vi "apply.graphic.filter.vi"(8 "error in (no error)":errorcluster, 10 "selection filter":T1={"Volume Type"={"Ongoing"=TRUE, "Limited Series"=TRUE, "Annuals"=TRUE, "One Shots"=TRUE, "Reference/Reprints"=TRUE, "Digital"=TRUE}, "team"=[], "characters"=[], "storyArcs"=[], "Plot End"=timestamp(0 s since 1904-01-01), "Plot Start"=timestamp(0 s since 1904-01-01), "title"=[], "colors"={"ongoing"=0, "Limited Series"=0, "Annuals"=0, "One Shots"=0, "Reprints"=0, "Digital"=0}, "concept"=[], "show all"=FALSE, "Search by Title"=enum."AND", "pub ids"=[]}, 11 "manager_daemon in":refnum<class "manager_daemon.lvclass">) -> (0 "error out":errorcluster, 3 "manager_daemon out":refnum<class "manager_daemon.lvclass">)   [LabVIEW 2024, in "manager_daemon.lvclass"]
uses:
  manager_daemon.lvclass
  TypeDefs/graphic.filter--cluster.ctl
  Graphic_UI/typedefs/volume.type.colors--cluster.ctl
  manager_daemon.lvclass/manager_daemon.ctl
  TypeDefs/issue.display--cluster.ctl
  CV_Shared_Library/volume.object--cluster.ctl
  CV_Shared_Library/volume.type--enum.ctl
  e2a5ae27-bb6a-44f0-90d7-e473ed9168d5.vi
  CV_Shared_Library/CV_Shared_Library.lvlib
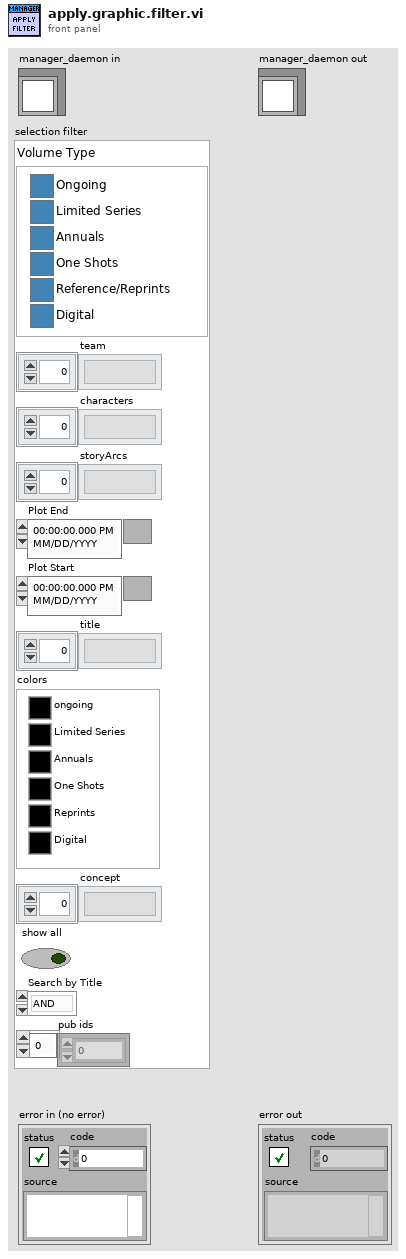
[diagram p1: front panel]
types:
  T1 = typedef "CV_Shared_Library.lvlib/graphic.filter--cluster.ctl" = cluster{"Volume Type":cluster{"Ongoing":bool, "Limited Series":bool, "Annuals":bool, "One Shots":bool, "Reference/Reprints":bool, "Digital":bool}, "team":string[], "characters":string[], "storyArcs":string[], "Plot End":timestamp, "Plot Start":timestamp, "title":string[], "colors":T2, "concept":string[], "show all":bool, "Search by Title":enum32{"AND", "OR"}, "pub ids":i32[]}
  T2 = typedef "volume.type.colors--cluster.ctl" = cluster{"ongoing":u32, "Limited Series":u32, "Annuals":u32, "One Shots":u32, "Reprints":u32, "Digital":u32}
  T3 = cluster{"Ongoing":bool, "Limited Series":bool, "Annuals":bool, "One Shots":bool, "Reference/Reprints":bool, "Digital":bool}
  T4 = typedef "manager_daemon.lvclass/IssueData--clustrer.ctl" = cluster{"cover_date":timestamp, "cv_id":string, "name":string, "sortable_name":string, "issue_number":string, "deck":string, "description":string, "volume id":i32, "store_date":timestamp, "date_last_updated":timestamp, "site_detail_url":string, "cover_url":string, "source_path":path, "in_collection":bool, "display_date":timestamp}
  T5 = typedef "manager_daemon.lvclass/sub-map--map.ctl" = map{string, T6}
  T6 = typedef "manager_daemon.lvclass/SubData--cluster.ctl" = cluster{"id":i32, "issues":set{i32}}
  T7 = typedef "manager_daemon.lvclass/VolumeData--cluster.ctl" = cluster{"name":string, "sortable_name":string, "aliases":string[], "description":string, "site_detail_url":string, "count_of_issues":i32, "start_year":i32, "publisher_id":i32, "issue_ids":i32[], "date_last_updated":timestamp, "volume":i32, "cv_id":string, "volume type":T8, "source_path":path}
  T8 = typedef "CV_Shared_Library.lvlib/volume.type--enum.ctl" = enum16{"Ongoing", "Limited Series", "Annual", "One Shot", "Reprint/Document", "Digital"}
  T9 = typedef "CV_Shared_Library.lvlib/volume.object--cluster.ctl" = cluster{"start date":timestamp, "end date":timestamp, "sortable_name":string, "color":u32, "volume type":T8, "issues":T10[]}
  T10 = typedef "CV_Shared_Library.lvlib/issue.display--cluster.ctl" = cluster{"cover_date":timestamp, "id":i32, "number":string, "fill":bool, "hilight":bool}
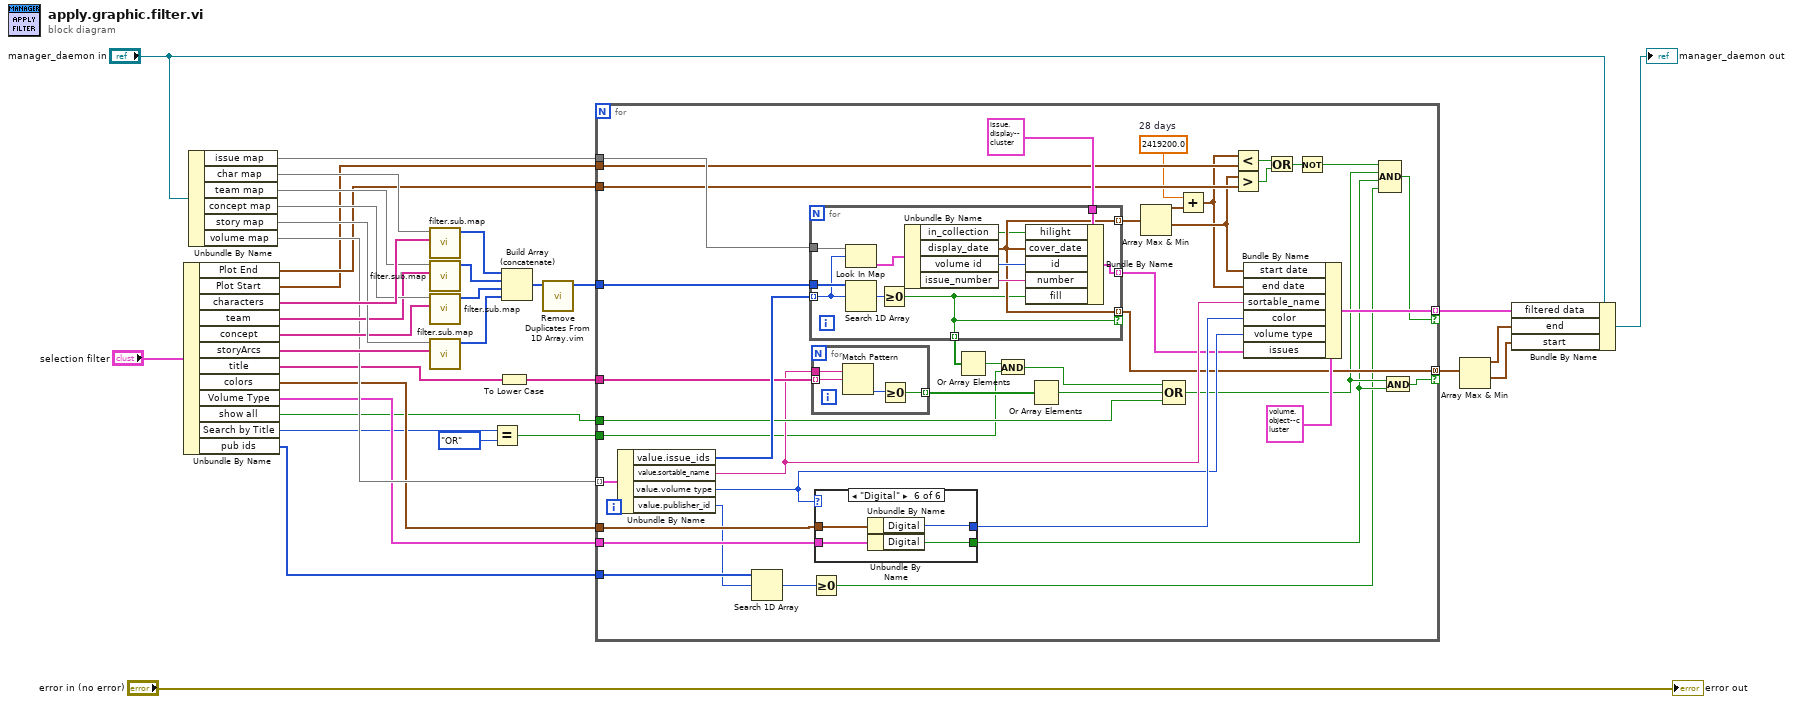
[diagram p0: block diagram]
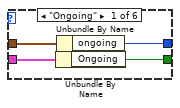
[diagram p2: hidden frame]
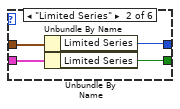
[diagram p3: hidden frame]
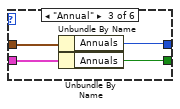
[diagram p4: hidden frame]
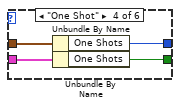
[diagram p5: hidden frame]
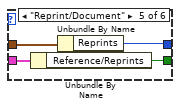
[diagram p6: hidden frame]
diagram:
  n1 = Unbundle By Name("selection filter") -> ("Plot End"=w14:timestamp, "Plot Start"=w13:timestamp, "characters"=w33:string[], "team"=w29:string[], "concept"=w28:string[], "storyArcs"=w27:string[], "title"=w19:string[], "colors"=w16:T2, "Volume Type"=w15:T3, "show all"=w12:bool, "Search by Title"=w7:enum32{"AND", "OR"}, "pub ids"=w1:i32[])
  n2 = Unbundle By Name("manager_daemon in") -> ("issue map"=w17:map{i32, T4}, "char map"=w34:T5, "team map"=w32:T5, "concept map"=w31:T5, "story map"=w30:T5, "volume map"=w26:map{i32, T7})
  n3 = call "filter.sub.map"("filter"=w33, "sub-map"=w34) -> ("issues"=w25:i32[])  [unwired: 9 in]
  n4 = call "filter.sub.map"("filter"=w29, "sub-map"=w32) -> ("issues"=w24:i32[])  [unwired: 9 in]
  n5 = call "filter.sub.map"("filter"=w28, "sub-map"=w31) -> ("issues"=w23:i32[])  [unwired: 9 in]
  n6 = call "filter.sub.map"("filter"=w27, "sub-map"=w30) -> ("issues"=w22:i32[])  [unwired: 9 in]
  n7 = Equal?(x=w7, y=enum32{"AND", "OR"}."OR") -> (x = y?=w5:bool)
  n8 = To Lower Case(string=w19) -> (all lower case string=w18:string[])
  n9 = Build Array (concatenate)(w25, w24, w23, w22) -> (w21:i32[])
  n10 = call "Remove Duplicates From 1D Array.vim"("array"=w21) -> ("array with duplicates removed"=w20:i32[])  [unwired: 10 in]
  n11 = for {
    tunnel: w26 -> [w76] mode=indexing
    tunnel: w20 -> [w74]
    tunnel: w18 -> [w72]
    tunnel: w17 -> [w73]
    tunnel: w16 -> [w69]
    tunnel: w15 -> [w68]
    tunnel: w14 -> [w64]
    tunnel: w13 -> [w65]
    tunnel: w12 -> [w60]
    tunnel: [w51] -> w9 mode=indexing if=w50
    tunnel: w5 -> [w45]
    tunnel: [w43] -> w4 mode=concatenating if=w42
    tunnel: w1 -> [w39]
    w49 = 2419200.0  # 28 days
    n12 = Unbundle By Name(w76) -> ("value.issue_ids"=w75:i32[], "value.sortable_name"=w55:string, "value.volume type"=w53:T8, "value.publisher_id"=w38:i32)
    n13 = Search 1D Array(1D array=w39, element=w38) -> (index of element=w37:i32)  [unwired: 1 in]
    n14 = for {
      tunnel: w75 -> [w114] mode=indexing
      tunnel: w74 -> [w115]
      tunnel: w73 -> [w116]
      tunnel: T10 {"cover_date"=timestamp(3329272800 s since 1904-01-01), "id"=162615, "number"="1", "fill"=TRUE, "hilight"=TRUE} ("issue") -> [w112]
      tunnel: [w108] -> w52 mode=indexing
      tunnel: [w107] -> w67 mode=indexing
      tunnel: [w106] -> w47 mode=indexing
      tunnel: [w107] -> w43 mode=indexing if=w106
      n15 = Look In Map(map=w116, key=w114) -> (value=w113:T4)  [unwired: 1 in, 1 out]
      n16 = Search 1D Array(1D array=w115, element=w114) -> (index of element=w109:i32)  [unwired: 1 in]
      n17 = Greater Or Equal To 0?(x=w109) -> (x >= 0?=w106:bool)
      n18 = Unbundle By Name(w113) -> ("in_collection"=w105:bool, "display_date"=w107:timestamp, "volume id"=w111:i32, "issue_number"=w110:string)
      n19 = Bundle By Name(cluster=w112, "hilight"=w105, "cover_date"=w107, "id"=w111, "number"=w110, "fill"=w106) -> (w108:T10)
    }
    n20 = Greater Or Equal To 0?(x=w37) -> (x >= 0?=w36:bool)
    n21 = for {
      tunnel: w72 -> [w103] mode=indexing
      tunnel: w55 -> [w104]
      tunnel: [w101] -> w71 mode=indexing
      n22 = Match Pattern(string=w104, regular expression=w103) -> (offset past match=w102:i32)  [unwired: 1 in, 3 out]
      n23 = Greater Or Equal To 0?(x=w102) -> (x >= 0?=w101:bool)
    }
    n24 = case shown="\"Digital\"" w53 {
      tunnel: w68 -> [w80 w84 w88 w92 w96 w100]
      tunnel: [w79 w83 w87 w91 w95 w99] -> w40
      tunnel: w69 -> [w78 w82 w86 w90 w94 w98]
      tunnel: [w77 w81 w85 w89 w93 w97] -> w54
      frame "Ongoing" {
        n25 = Unbundle By Name(w80) -> ("Ongoing"=w79:bool)
        n26 = Unbundle By Name(w78) -> ("ongoing"=w77:u32)
      }
      frame "Limited Series" {
        n27 = Unbundle By Name(w82) -> ("Limited Series"=w81:u32)
        n28 = Unbundle By Name(w84) -> ("Limited Series"=w83:bool)
      }
      frame "Annual" {
        n29 = Unbundle By Name(w86) -> ("Annuals"=w85:u32)
        n30 = Unbundle By Name(w88) -> ("Annuals"=w87:bool)
      }
      frame "One Shot" {
        n31 = Unbundle By Name(w90) -> ("One Shots"=w89:u32)
        n32 = Unbundle By Name(w92) -> ("One Shots"=w91:bool)
      }
      frame "Reprint/Document" {
        n33 = Unbundle By Name(w96) -> ("Reference/Reprints"=w95:bool)
        n34 = Unbundle By Name(w94) -> ("Reprints"=w93:u32)
      }
      frame "Digital" {
        n35 = Unbundle By Name(w98) -> ("Digital"=w97:u32)
        n36 = Unbundle By Name(w100) -> ("Digital"=w99:bool)
      }
    }
    n37 = Or Array Elements(Boolean array=w47) -> (logical OR=w46:bool)
    n38 = And(x=w46, y=w45) -> (x .and. y?=w44:bool)
    n39 = Or Array Elements(Boolean array=w71) -> (logical OR=w48:bool)
    n40 = Array Max & Min(array=w67) -> (max value=w66:timestamp, min value=w57:timestamp)  [unwired: 2 out]
    n41 = Compound Arithmetic op=OR(w44, w48, w60) -> (w41:bool)
    n42 = Add(x=w49, y=w66) -> (x+y=w56:timestamp)
    n43 = Less?(x=w56, y=w65) -> (x < y?=w62:bool)
    n44 = Greater?(x=w57, y=w64) -> (0:w61:bool)
    n45 = Bundle By Name(cluster=T9 {"start date"=timestamp(0 s since 1904-01-01), "end date"=timestamp(0 s since 1904-01-01), "sortable_name"="", "color"=0, "volume type"=enum."Ongoing", "issues"=[]} ("Cluster"), "start date"=w57, "end date"=w56, "sortable_name"=w55, "color"=w54, "volume type"=w53, "issues"=w52) -> (w51:T9)
    n46 = Or(x=w62, y=w61) -> (x .or. y?=w63:bool)
    n47 = Not(x=w63) -> (.not. x?=w59:bool)
    n48 = Compound Arithmetic op=AND(w59, w41, w40, w36) -> (w50:bool)
    n49 = And(x=w41, y=w40) -> (x .and. y?=w42:bool)
  }
  n50 = Array Max & Min(array=w4) -> (max value=w3:timestamp, min value=w2:timestamp)  [unwired: 2 out]
  n51 = Bundle By Name(cluster="manager_daemon in", "filtered data"=w9, "end"=w3, "start"=w2) -> (→"manager_daemon out":refnum<class "manager_daemon.lvclass">)
  "error out" <- "error in (no error)"
